vi "Destroy.vi"(11 "jettl Queue Actor in":refnum<class "jettl Queue Actor.lvclass">) -> (3 "jettl Queue Actor out":refnum<class "jettl Queue Actor.lvclass">)   [LabVIEW 2021, in "jettl.lvlib" / "jettl Queue Actor.lvclass"]
uses:
  jettl Queue Actor.lvclass
  jettl Queue Actor.lvclass/jettl Queue Actor.ctl
  Actor/Msgs/Last Ack/Last Ack Msg/Last Ack Msg.lvclass
  C:/git/jettl/src/Actor/Msg/Msg.lvclass
  jettl.lvlib
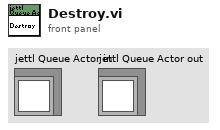
[diagram p1: front panel]
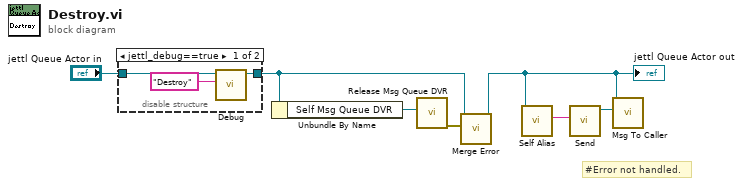
[diagram p0: block diagram]
diagram:
  # "#Error not handled."
  n1 = disable-structure shown="jettl_debug==true" {
    disable-tunnel: "jettl Queue Actor in" -> [w10 w11]
    disable-tunnel: [w9 w11] -> w2
    frame condition #0 (active) {
      n2 = call "Debug.vi"("Method"="Destroy", "jettl Queue Actor in"=w10) -> ("jettl Queue Actor out"=w9:refnum<class "jettl Queue Actor.lvclass">)  [unwired: 9 in]
    }
    frame condition #1 {
    }
  }
  n3 = Unbundle By Name(w2) -> ("Self Msg Queue DVR"=w4:refnum<data-value>)
  n4 = call "Release Msg Queue DVR.vi"("Msg Queue DVR"=w4) -> ("error out"=w3:errorcluster)  [unwired: 10 in]
  n5 = call-dynamic "Merge Error.vi"("Error"=w3, "jettl Queue Actor in"=w2) -> ("jettl Queue Actor out"=w1:refnum<class "jettl Queue Actor.lvclass">)  [unwired: 9 in]
  "jettl Queue Actor out" <- w1
  n6 = call-dynamic "Self Alias.vi"("jettl Queue Actor in"=w1) -> ("Self Alias"=w5:string)  [unwired: 10 in]
  n7 = call "Send.vi"("Alias"=w5) -> ("Last Ack Msg out"=w7:refnum<class "Last Ack Msg.lvclass">)  [unwired: 10 in]
  n8 = call-dynamic "Msg To Caller.vi"("Msg"=w7, "jettl Queue Actor in"=w1) -> ()  [unwired: 9 in, 1 out]
